vi "write_hardware_seqs.vi"(8 "error in (no error)":errorcluster, 10 "hardware_SEQs":T1, 11 "panel in":refnum<class "panel.lvclass">) -> (0 "error out":errorcluster, 3 "panel out":refnum<class "panel.lvclass">)   [LabVIEW 2015, in "panel.lvclass"]
uses:
  panel.lvclass
  front_panel_class/hardware_seqs.ctl
  Hardware Class/hardware/hardware.lvclass
  panel.lvclass/panel.ctl
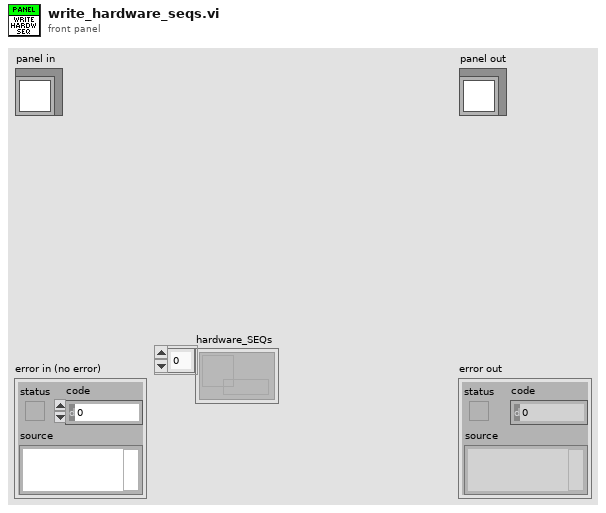
[diagram p1: front panel]
types:
  T1 = typedef "hardware_seqs.ctl" = refnum<queue>[]
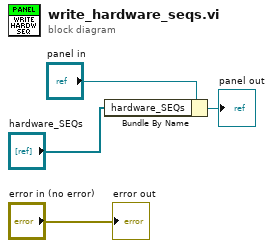
[diagram p0: block diagram]
diagram:
  n1 = Bundle By Name(cluster="panel in", "hardware_SEQs"="hardware_SEQs") -> (→"panel out":refnum<class "panel.lvclass">)
  "error out" <- "error in (no error)"
